vi "AB_Engine_DLL_Verify_ProtoDefined.vi"(4 "compatabilityWIth2011":bool=TRUE, 6 "destinations":refnum<class "AB_Destination.lvclass">[](array[class]), 7 "path":path, 8 "error in (no error)":errorcluster, 10 "flat file layout":bool, 11 "sourceItems":refnum<class "AB_Source.lvclass">[](array[class])) -> (0 "error out":errorcluster, 1 "vipInfo":T1[](array[typedef]), 2 "viNames":string[](array[string]))   [LabVIEW 2020]
uses:
  <vilib>/AppBuilder/AB_Classes/Source/AB_Source.lvclass
  <vilib>/AppBuilder/ABAPI Dist VI Proto Info New.ctl
  <vilib>/AppBuilder/AB_Classes/Destination/AB_Destination.lvclass
  <vilib>/AppBuilder/AB_Classes/Source/ExportedVI/AB_Source_ExportedVI.lvclass
  <resource>/Framework/Providers/Common/provcom_StringGlobals.vi
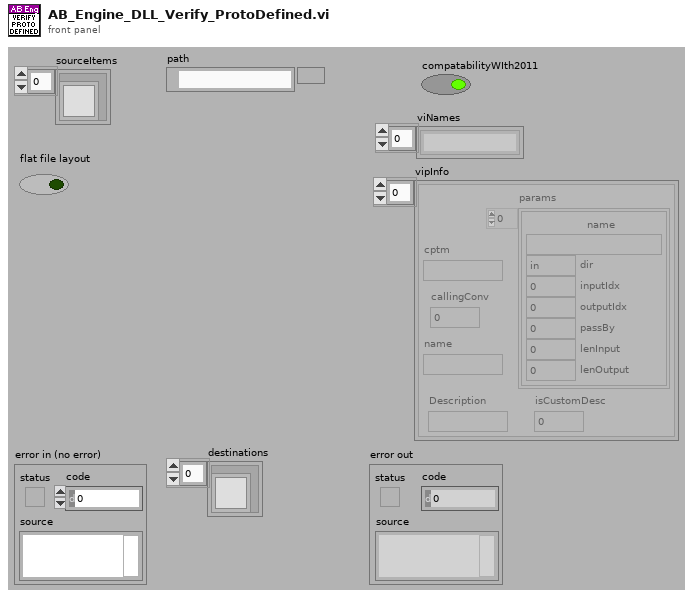
[diagram p1: front panel]
types:
  T1 = typedef "ABAPI Dist VI Proto Info New.ctl" = cluster{"cptm":string, "params":cluster{"name":string, "dir":enum32{"in", "out", "in/out", "length", "error-out"}, "inputIdx":i32, "outputIdx":i32, "passBy":i32, "lenInput":i32, "lenOutput":i32}[], "callingConv":i32, "name":string, "Description":string, "isCustomDesc":i32}
  T2 = typedef "AB_Source.ctl" = cluster{"path":path, "itemID":string, "parentIndex":i32, "sourceInclusion":T3, "destinationIndex":i32, "properties":T4[], "newName":string, "lvfile":bool, "valid":bool, "eng_inBuild":bool, "eng_isNonVILink":bool, "Amalgamation":bool, "Amalgamation Piece":bool, "eng_delimitedName":string, "preventRename":bool}
  T3 = typedef "AB_Source_Inclusion.ctl" = enum16{"IncludeIfReferenced", "Include", "Exclude", "TopLevel"}
  T4 = typedef "AB_Source_Properties.ctl" = cluster{"sourcePropertyType":T5, "value":variant}
  T5 = typedef "AB_Source_Property_Type.ctl" = enum16{"Remove block diagram", "Remove front panel", "Password", "Window has title bar", "Show menu bar", "Show vertical scroll bar", "Show horizontal scroll bar", "Show toolbar", "Show Abort button", "Show fp when called", "Window behavior", "Allow user to close window", "Window run-time position", "Run when opened", "Allow debugging", "Auto error handling", "Generate guard code", "Use stack variables", "Expression folding", "Integer only", "Inline subVI"}
  T6 = typedef "AB_Destination.ctl" = cluster{"destName":string, "path":path, "libraryName":string, "preserveHierarchy":bool, "eng_inBuild":bool, "eng_libraryReference":refnum<vi>, "eng_restictAddToNewLibrary":bool}
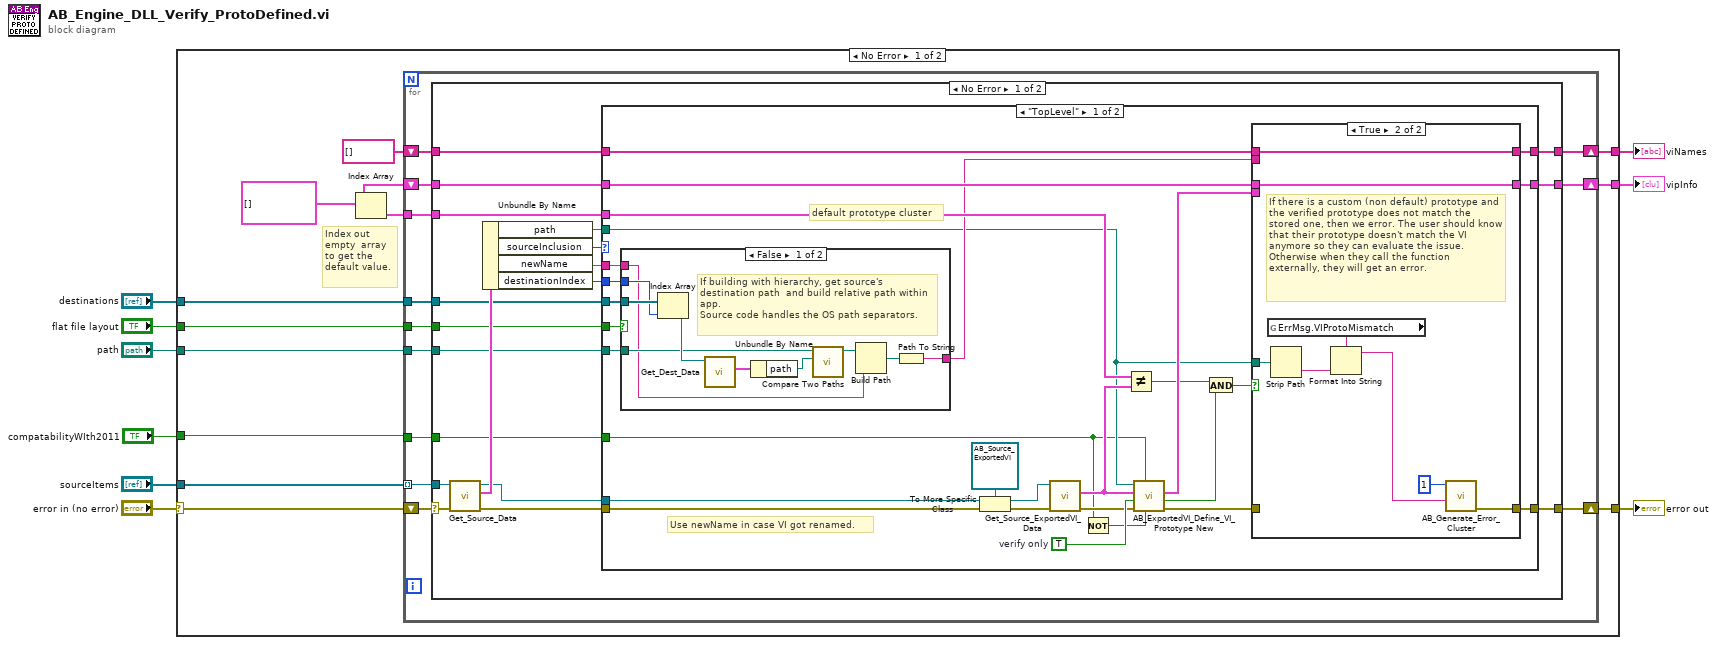
[diagram p0: block diagram]
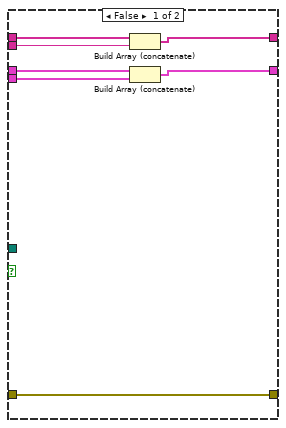
[diagram p2: hidden frame]
diagram:
  n1 = case shown="No Error" "error in (no error)" {
    selector: "error in (no error)" -> [w20 w113]
    tunnel: [w19 w113] -> w8
    tunnel: "sourceItems" -> [w21 _]
    tunnel: [w17 _] -> w6
    tunnel: [w16 _] -> w5
    tunnel: "flat file layout" -> [w15 _]
    tunnel: "destinations" -> [w14 _]
    tunnel: "path" -> [w13 _]
    tunnel: "compatabilityWIth2011" -> [w10 _]
    frame No Error {
      w12 = T1[] []
      # "Index out empty  array to get the default value."
      n2 = Index Array(array=w12) -> (element=w11:T1)  [unwired: 1 in]
      n3 = for {
        tunnel: w21 -> [w33] mode=indexing
        shift-right: [w32] -> w19
        shift-left: w20 -> [w31]
        shift-right: [w28] -> w17
        shift-left: string[] [] -> [w27]
        shift-right: [w30] -> w16
        shift-left: w12 -> [w29]
        tunnel: w15 -> [w26]
        tunnel: w14 -> [w25]
        tunnel: w13 -> [w24]
        tunnel: w11 -> [w23]
        tunnel: w10 -> [w22]
        n4 = case shown="No Error" w31 {
          selector: w31 -> [w46 w112]
          tunnel: w33 -> [w49 _]
          tunnel: [w47 w112] -> w32
          tunnel: [w45 w110] -> w30
          tunnel: w29 -> [w44 w110]
          tunnel: [w43 w111] -> w28
          tunnel: w27 -> [w42 w111]
          tunnel: w26 -> [w41 _]
          tunnel: w25 -> [w38 _]
          tunnel: w24 -> [w37 _]
          tunnel: w23 -> [w35 _]
          tunnel: w22 -> [w34 _]
          frame No Error {
            n5 = call <vilib>:"Get_Source_Data.vi"("error in (no error)"=w46, "Class in"=w49) -> ("error out"=w48:errorcluster, "data"=w52:T2, "Class out"=w50:refnum<class "AB_Source.lvclass">)  [unwired: 7 out]
            n6 = Unbundle By Name(w52) -> ("path"=w36:path, "sourceInclusion"=w51:T3, "newName"=w40:string, "destinationIndex"=w39:i32)
            n7 = case shown="\"TopLevel\"" w51 {
              tunnel: w36 -> [w56 _]
              tunnel: w50 -> [w79 _]
              tunnel: w48 -> [w73 w109]
              tunnel: [w62 w109] -> w47
              tunnel: [w77 w107] -> w45
              tunnel: w44 -> [w76 w107]
              tunnel: [w75 w108] -> w43
              tunnel: w42 -> [w74 w108]
              tunnel: w41 -> [w71 _]
              tunnel: w40 -> [w70 _]
              tunnel: w39 -> [w67 _]
              tunnel: w38 -> [w69 _]
              tunnel: w37 -> [w68 _]
              tunnel: w35 -> [w64 _]
              tunnel: w34 -> [w53 _]
              frame "TopLevel" {
                w78 = TRUE  # verify only
                # "default prototype cluster"
                # "Use newName in case VI got renamed."
                n8 = case shown="False" w71 {
                  tunnel: w70 -> [w98 w106]
                  tunnel: [w96 w106] -> w57
                  tunnel: w69 -> [w105 _]
                  tunnel: w68 -> [w101 _]
                  tunnel: w67 -> [w104 _]
                  frame False {
                    # "If building with hierarchy, get source's destination path  and build relative path within app. \nSource code handles the OS path separators."
                    n9 = Index Array(array=w105, index=w104) -> (element=w103:refnum<class "AB_Destination.lvclass">)
                    n10 = call <vilib>:"Get_Dest_Data.vi"("Class in"=w103) -> ("destName"=w102:T6)  [unwired: 1 in, 9 out]
                    n11 = Unbundle By Name(w102) -> ("path"=w100:path)
                    n12 = call <vilib>:"Compare Two Paths.vi"("Path 2"=w100, "Path 1"=w101) -> ("Relative Path from 1 to 2"=w99:path)  [unwired: 1 in, 8 out]
                    n13 = Build Path(base path=w99, name or relative path=w98) -> (appended path=w97:path)
                    n14 = Path To String(path=w97) -> (string=w96:string)
                  }
                  frame True {
                    # "If building in a flat format (i.e. using LLBs or compatibility mode), just pass through VI's new name."
                  }
                }
                n15 = To More Specific Class(target class=refnum<class "AB_Source_ExportedVI.lvclass"> refnum ("Class in"), reference=w79, error in=w73) -> (specific class reference=w66:refnum<class "AB_Source_ExportedVI.lvclass">, error out=w65:errorcluster)
                n16 = call <vilib>:"Get_Source_ExportedVI_Data.vi"("error in (no error)"=w65, "Class in"=w66) -> ("error out"=w72:errorcluster, "data"=w61:T1)  [unwired: 8 out]
                n17 = Not(x=w53) -> (.not. x?=w54:bool)
                n18 = Not Equal?(x=w64, y=w61) -> (x != y?=w59:bool)
                n19 = call <vilib>:"AB_ExportedVI_Define_VI_Prototype New.vi"("generateNamespace"=w54, "compatibilityMode"=w53, "error in (no error)"=w72, "verify only"=w78, "vipInfo in"=w61, "path"=w56) -> ("error out"=w63:errorcluster, "cptmMismatch"=w55:bool, "vipInfo out"=w60:T1)  [unwired: 3 in]
                n20 = And(x=w59, y=w55) -> (x .and. y?=w58:bool)
                n21 = case shown="True" w58 {
                  tunnel: [w87 w94] -> w77
                  tunnel: w76 -> [w86 w94]
                  tunnel: [w85 w95] -> w75
                  tunnel: w74 -> [w84 w95]
                  tunnel: w57 -> [w83 _]
                  tunnel: w60 -> [w82 _]
                  tunnel: w63 -> [w81 _]
                  tunnel: [w81 w93] -> w62
                  tunnel: w56 -> [_ w91]
                  frame False {
                    n22 = Build Array (concatenate)(w84, w83) -> (w85:string[])
                    n23 = Build Array (concatenate)(w86, w82) -> (w87:T1[])
                  }
                  frame True {
                    # "If there is a custom (non default) prototype and the verified prototype does not match the stored one, then we error. The user should know that their prototype doesn't match the VI anymore so they can evaluate the issue. Otherwise when they call the function externally, they will get an error."
                    n24 = global read "provcom_StringGlobals.vi" "ErrMsg.VIProtoMismatch"() -> (w90:string)
                    n25 = Strip Path(path=w91) -> (name=w89:string)  [unwired: 1 out]
                    n26 = Format Into String(format string=w90, w89) -> (resulting string=w88:string)  [unwired: 2 in, 1 out]
                    n27 = call <vilib>:"AB_Generate_Error_Cluster.vi"("Additional Message"=w88, "Code"=1) -> ("error out"=w93:errorcluster)  [unwired: 2 in, 7 out]
                  }
                }
              }
              frame Default {
              }
            }
          }
          frame Error {
          }
        }
      }
    }
    frame Error {
    }
  }
  "error out" <- w8
  "viNames" <- w6
  "vipInfo" <- w5
